vi "_ast_example.vi"() -> ()   [LabVIEW 2017]
uses:
  ast_db.vi
  ast_table_list.vi
panel:
  out "token":u64 format="%016x"
  out "query":string
  out "error out":errorcluster
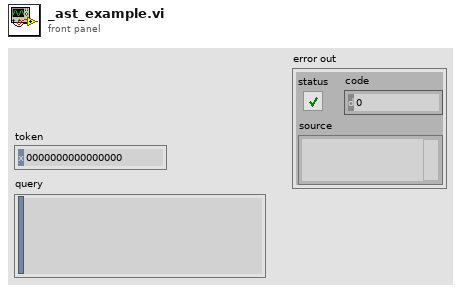
[diagram p1: front panel]
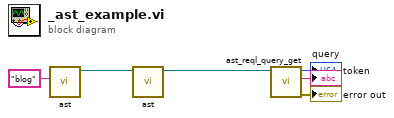
[diagram p0: block diagram]
diagram:
  n1 = call-poly "ast.vi"("db_name"="blog") -> ("db"=w6:refnum<k1>)  [unwired: 10 in]
  n2 = call-poly "ast.vi"("db"=w6) -> ("table"=w5:refnum<k1>)  [unwired: 10 in]
  n3 = call "ast_reql_query_get.vi"("query_id in"=w5) -> ("error out"=→"error out":errorcluster, "query"=→"query":string, "query_id out"=→"token":u32)  [unwired: 8 in]
